vi "NicmosMaskGenerator.vi"(2 "MASKBANKS":T1, 9 "error in (no error)":errorcluster caption="entrée d'erreur") -> (0 "Mask List":bool[][][](array[boolean]), 6 "error out":errorcluster caption="sortie d'erreur")   [LabVIEW 2009]
uses:
  Controls/NICMOS.MASKBANKS.ctl
  NicmosGlobal.vi
panel:
  out "Bank 7":i16[][](graph)
  out "Bank 6":i16[][](graph)
  out "Bank 5":i16[][](graph)
  out "Bank 4":i16[][](graph)
  out "Bank 3":i16[][](graph)
  out "Bank 2":i16[][](graph)
  out "Bank 1":i16[][](graph)
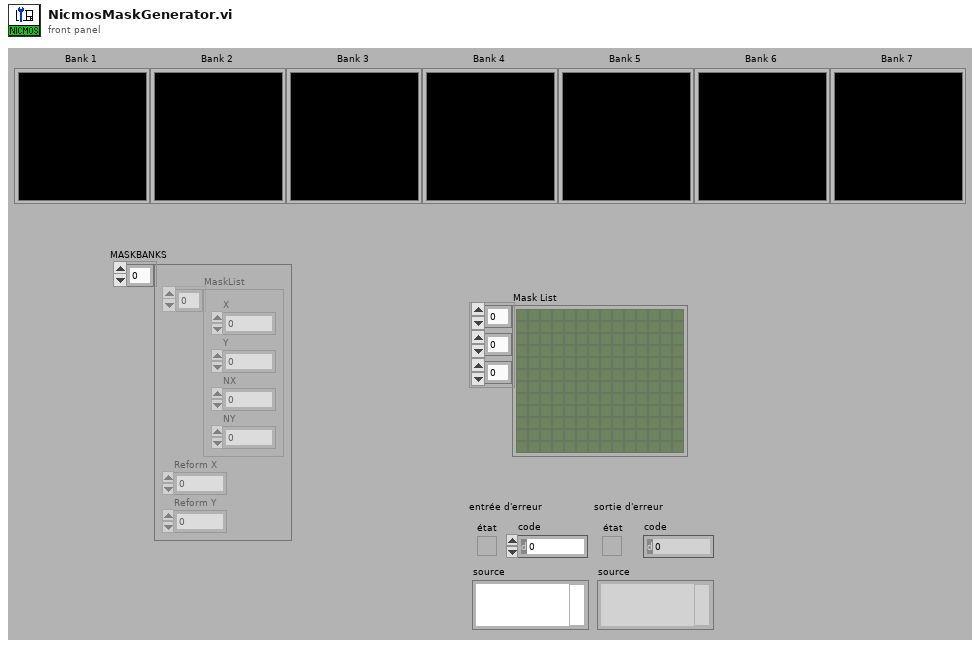
[diagram p1: front panel]
types:
  T1 = typedef "NICMOS.MASKBANKS.ctl" = cluster{"MaskList":cluster{"X":i32, "Y":i32, "NX":i32, "NY":i32}[], "Reform X":i32, "Reform Y":i32}[]
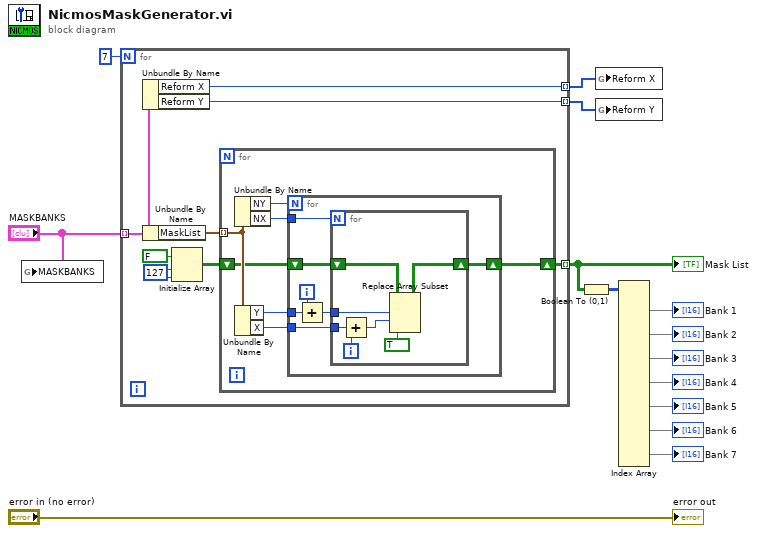
[diagram p0: block diagram]
diagram:
  n1 = global write "NicmosGlobal.vi" "MASKBANKS"("MASKBANKS") -> ()
  n2 = for {
    N: 7 -> [_]
    tunnel: "MASKBANKS" -> [w17] mode=indexing
    tunnel: [w18] -> w13 mode=indexing
    tunnel: [w16] -> w2 mode=indexing
    tunnel: [w15] -> w1 mode=indexing
    w20 = 127 ("taille de la dimension")
    n3 = Unbundle By Name(w17) -> ("Reform X"=w16:i32, "Reform Y"=w15:i32)
    n4 = Unbundle By Name(w17) -> ("MaskList"=w22:cluster{"X":i32, "Y":i32, "NX":i32, "NY":i32}[])
    n5 = Initialize Array(FALSE ("élément"), w20, w20) -> (w19:bool[][])
    n6 = for {
      tunnel: w22 -> [w27] mode=indexing
      shift-right: [w23] -> w18
      shift-left: w19 -> [w24]
      n7 = Unbundle By Name(w27) -> ("NY"=w29:i32, "NX"=w28:i32)
      n8 = Unbundle By Name(w27) -> ("Y"=w26:i32, "X"=w25:i32)
      n9 = for {
        N: w29 -> [_]
        tunnel: w28 -> [w36]
        tunnel: w26 -> [w34]
        tunnel: w25 -> [w33]
        shift-right: [w30] -> w23
        shift-left: w24 -> [w31]
        i -> [w35]
        n10 = Add(x=w34, y=w35) -> (x+y=w32:i32)
        n11 = for {
          N: w36 -> [_]
          tunnel: w33 -> [w42]
          tunnel: w32 -> [w40]
          shift-right: [w37] -> w30
          shift-left: w31 -> [w41]
          i -> [w43]
          n12 = Add(x=w42, y=w43) -> (x+y=w39:i32)
          n13 = Replace Array Subset(array=w41, new element=TRUE ("nouvel élt/sous-tableau"), index (row)=w40, index (col)=w39) -> (w37:bool[][])
        }
      }
    }
  }
  "Mask List" <- w13
  n14 = Boolean To (0,1)(Boolean=w13) -> (0, 1=w12:i16[][][])
  n15 = global write "NicmosGlobal.vi" "Reform X"(w2) -> ()
  n16 = global write "NicmosGlobal.vi" "Reform Y"(w1) -> ()
  n17 = Index Array(array=w12) -> (element #1=→"Bank 1":i16[][], element #2=→"Bank 2":i16[][], element #3=→"Bank 3":i16[][], element #4=→"Bank 4":i16[][], element #5=→"Bank 5":i16[][], element #6=→"Bank 6":i16[][], element #7=→"Bank 7":i16[][])  [unwired: 21 in]
  "error out" <- "error in (no error)"
